vi "RichToFlatnixnet_grpc_StatusToStringResponse.vi"(5 "OutputClusterType":T1, 11 "InputCluster":T2) -> (3 "OutputCluster":T1)   [LabVIEW 2025, in "xnet-grpc_client.lvlib"]
uses:
  nixnet_grpc_StatusToStringResponse.ctl
  nixnet_grpc_StatusToStringResponse_Flat.ctl
  xnet-grpc_client.lvlib
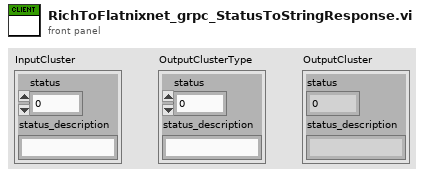
[diagram p1: front panel]
types:
  T1 = typedef "xnet-grpc_client.lvlib/nixnet_grpc_StatusToStringResponse_Flat.ctl" = cluster{"status":i32, "status_description":string}
  T2 = typedef "xnet-grpc_client.lvlib/nixnet_grpc_StatusToStringResponse.ctl" = cluster{"status":i32, "status_description":string}
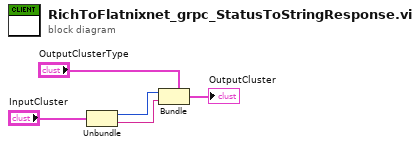
[diagram p0: block diagram]
diagram:
  n1 = Unbundle "Unbundle"("InputCluster") -> ("status"=w2:i32, "status_description"=w1:string)
  n2 = Bundle "Bundle"(cluster="OutputClusterType", "status"=w2, "status_description"=w1) -> (→"OutputCluster":T1)
